vi "plot lines.vi"(0 "P1x":dbl[](array[numeric])=[0.0, -5.0, -5.0], 1 "P1y":dbl[](array[numeric])=[0.0, 5.0, 10.0], 2 "P2x":dbl[](array[numeric])=[10.0, 5.0, 5.0], 3 "P2y":dbl[](array[numeric])=[10.0, 5.0, -10.0], 4 "dL":dbl=0.5) -> (5 "LX":dbl[](array[numeric]), 6 "LY":dbl[](array[numeric]))   [LabVIEW 2009]
panel:
  out "XY Graph":cluster{dbl[], dbl[]}(graph)
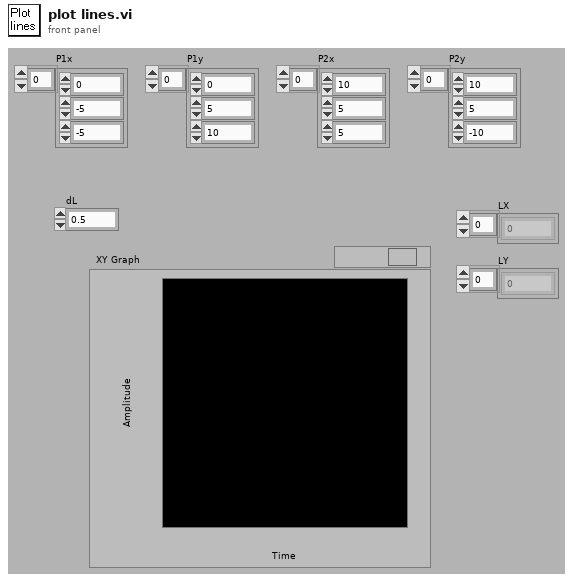
[diagram p1: front panel]
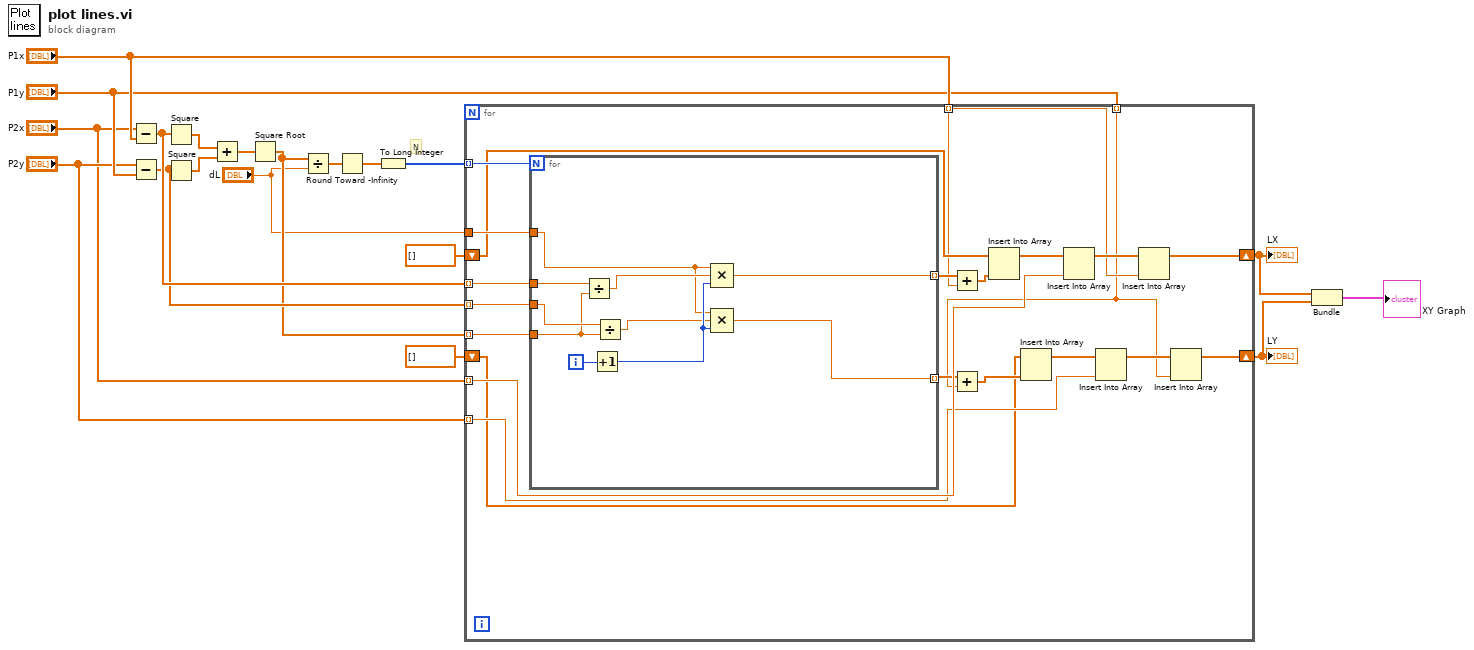
[diagram p0: block diagram]
diagram:
  # "N"
  n1 = Subtract(x="P2x", y="P1x") -> (x-y=w13:dbl[])
  n2 = Subtract(x="P2y", y="P1y") -> (x-y=w12:dbl[])
  n3 = Square(x=w13) -> (x^2=w19:dbl[])
  n4 = Square(x=w12) -> (x^2=w18:dbl[])
  n5 = Add(x=w19, y=w18) -> (x+y=w17:dbl[])
  n6 = Square Root(x=w17) -> (sqrt(x)=w11:dbl[])
  n7 = Divide(x=w11, y="dL") -> (x/y=w16:dbl[])
  n8 = Round Toward -Infinity(1:w16) -> (0:w15:dbl[])
  n9 = To Long Integer(number=w15) -> (32bit integer=w14:i32[])
  n10 = for {
    tunnel: w14 -> [w40] mode=indexing
    tunnel: "P2x" -> [w30] mode=indexing
    tunnel: "P2y" -> [w26] mode=indexing
    tunnel: w13 -> [w39] mode=indexing
    tunnel: w12 -> [w38] mode=indexing
    tunnel: w11 -> [w37] mode=indexing
    tunnel: "dL" -> [w36]
    shift-right: [w34] -> w5
    shift-left: dbl[] [] -> [w35]
    tunnel: "P1x" -> [w21] mode=indexing
    tunnel: "P1y" -> [w20] mode=indexing
    shift-right: [w23] -> w4
    shift-left: dbl[] [] -> [w22]
    n11 = for {
      N: w40 -> [_]
      tunnel: w39 -> [w49]
      tunnel: w38 -> [w48]
      tunnel: w37 -> [w47]
      tunnel: w36 -> [w43]
      tunnel: [w42] -> w31 mode=indexing
      tunnel: [w41] -> w27 mode=indexing
      i -> [w50]
      n12 = Divide(x=w49, y=w47) -> (x/y=w46:dbl)
      n13 = Increment(x=w50) -> (x+1=w45:i32)
      n14 = Divide(x=w48, y=w47) -> (x/y=w44:dbl)
      n15 = Compound Arithmetic op=MULTIPLY(w43, w46, w45) -> (w42:dbl)
      n16 = Compound Arithmetic op=MULTIPLY(w43, w44, w45) -> (w41:dbl)
    }
    n17 = Add(x=w31, y=w21) -> (x+y=w29:dbl[])
    n18 = Add(x=w27, y=w20) -> (x+y=w28:dbl[])
    n19 = Insert Into Array(array=w35, new element=w29) -> (w32:dbl[])  [unwired: 1 in]
    n20 = Insert Into Array(array=w22, new element=w28) -> (w25:dbl[])  [unwired: 1 in]
    n21 = Insert Into Array(array=w32, new element=w30) -> (w33:dbl[])  [unwired: 1 in]
    n22 = Insert Into Array(array=w25, new element=w26) -> (w24:dbl[])  [unwired: 1 in]
    n23 = Insert Into Array(array=w33, new element=w21) -> (w34:dbl[])  [unwired: 1 in]
    n24 = Insert Into Array(array=w24, new element=w20) -> (w23:dbl[])  [unwired: 1 in]
  }
  "LX" <- w5
  "LY" <- w4
  n25 = Bundle(w5, w4) -> (→"XY Graph":cluster{dbl[], dbl[]})  [unwired: 1 in]
